vi "SetParam.vi"(8 "error in (no error)":errorcluster caption="entrée d'erreur (pas d'erreur)", 10 "johnson_lindenstrauss_min_dim":cluster{"n_samples":i32[], "eps":dbl[]} {"eps" min=0.0 max=1.0}, 11 "Johnson_lindenstrauss_min_dim.lvclass":refnum<class "Johnson_lindenstrauss_min_dim.lvclass">) -> (0 "error out":errorcluster caption="sortie d'erreur", 3 "Johnson_lindenstrauss_min_dim.lvclass":refnum<class "Johnson_lindenstrauss_min_dim.lvclass">)   [LabVIEW 2020, in "Johnson_lindenstrauss_min_dim.lvclass"]
doc: "Set Parameters"
uses:
  Johnson_lindenstrauss_min_dim.lvclass
  Johnson_lindenstrauss_min_dim.lvclass/Johnson_lindenstrauss_min_dim.ctl
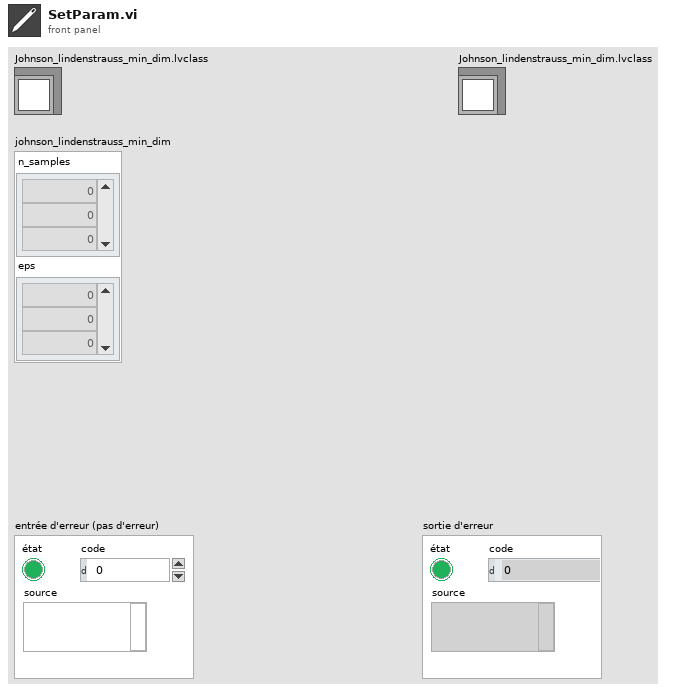
[diagram p1: front panel]
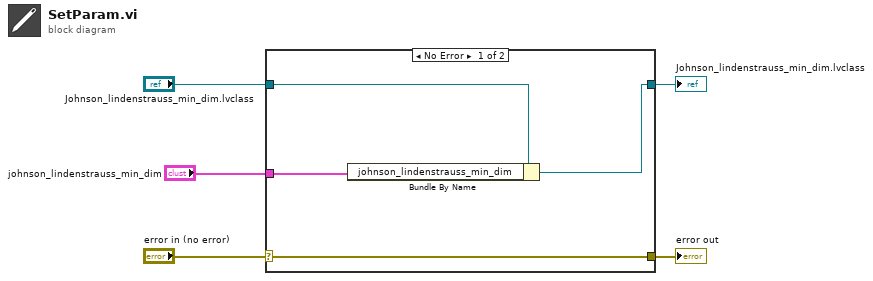
[diagram p0: block diagram]
diagram:
  n1 = case shown="No Error" "error in (no error)" {
    selector: "error in (no error)" -> [w9 w10]
    tunnel: [w9 w10] -> w4
    tunnel: [w7 w11] -> w2
    tunnel: "Johnson_lindenstrauss_min_dim.lvclass" -> [w8 w11]
    tunnel: "johnson_lindenstrauss_min_dim" -> [w6 _]
    frame No Error {
      n2 = Bundle By Name(cluster=w8, "johnson_lindenstrauss_min_dim"=w6) -> (w7:refnum<class "Johnson_lindenstrauss_min_dim.lvclass">)
    }
    frame Error {
    }
  }
  "error out" <- w4
  "Johnson_lindenstrauss_min_dim.lvclass" <- w2
